vi "Camera Direction Control.vi"(1 "Current Driving Direction (True = Shooter Forward)":bool, 2 "Camera Switch":bool) -> (0 "Camera Direction (True = Shooter Camera)":bool)   [LabVIEW 2015]
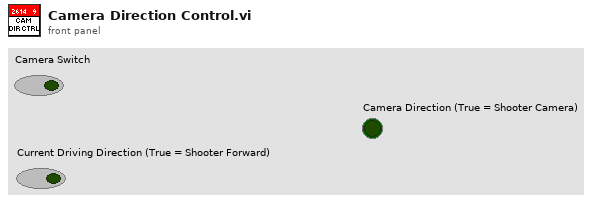
[diagram p1: front panel]
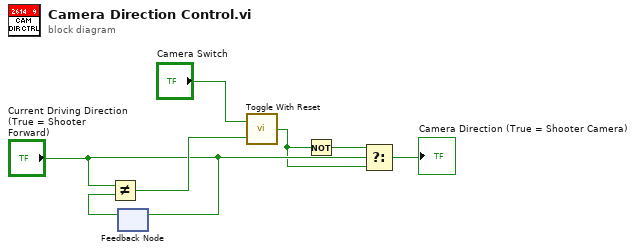
[diagram p0: block diagram]
diagram:
  n1 = feedback-in #1("Current Driving Direction (True = Shooter Forward)") -> ()
  n2 = feedback #1() -> (w7:bool)  [unwired: 1 in]
  n3 = Not Equal?(x="Current Driving Direction (True = Shooter Forward)", y=w7) -> (x != y?=w6:bool)
  n4 = call "Toggle With Reset.vi"("Reset"=w6, "Boolean"="Camera Switch") -> ("Driver Switch 2"=w3:bool)
  n5 = Not(x=w3) -> (.not. x?=w1:bool)
  n6 = Select(t=w1, s="Current Driving Direction (True = Shooter Forward)", f=w3) -> (s? t:f=→"Camera Direction (True = Shooter Camera)":bool)
